vi "navX_SPI_CRC.vi"(0 "Message":u8[](array[numeric])=[255, 43, 176, 52, 27, 0, 240]) -> (1 "Message with CRC":u8[](array[numeric]), 2 "CRC":u8 format="%.0x")   [LabVIEW 2016]
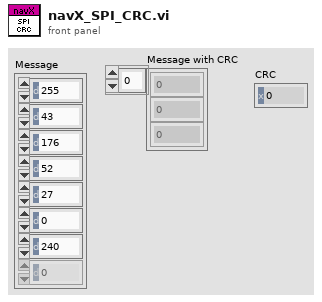
[diagram p1: front panel]
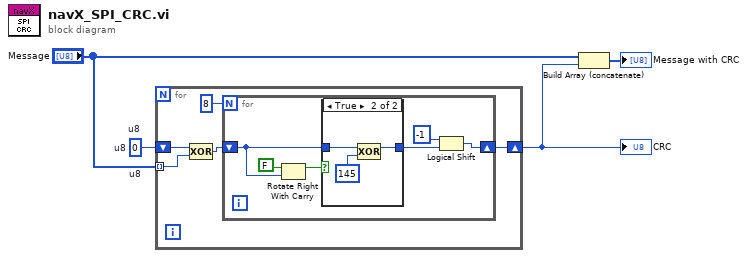
[diagram p0: block diagram]
diagram:
  w1 = u8 0  # u8
  (unwired) u8 0  # u8
  (unwired) u8 0  # u8
  n1 = for {
    shift-right: [w6] -> w3
    shift-left: w1 -> [w9]
    tunnel: "Message" -> [w7] mode=indexing
    n2 = Compound Arithmetic op=XOR(w9, w7) -> (w5:u8)
    n3 = for {
      N: 8 -> [_]
      shift-right: [w14] -> w6
      shift-left: w5 -> [w11]
      n4 = Rotate Right With Carry(2:w11, 3:FALSE ("carry")) -> (1:w12:bool)  [unwired: 1 out]
      n5 = case shown="True" w12 {
        tunnel: [w16 w18] -> w15
        tunnel: w11 -> [w16 w19]
        frame False {
        }
        frame True {
          n6 = Compound Arithmetic op=XOR(w19, u8 145 ("value")) -> (w18:u8)
        }
      }
      n7 = Logical Shift(y=i16 -1, x=w15) -> (x << y=w14:u8)
    }
  }
  "CRC" <- w3
  n8 = Build Array (concatenate)("Message", w3) -> (→"Message with CRC":u8[])
